vi "Is Already Exists.vi"(10 "Error":errorcluster) -> (2 "Error":errorcluster)   [LabVIEW 2020, in "jettl.lvlib" / "Actor.lvlib"]
uses:
  Actor.lvlib
  Error/Error.lvlib
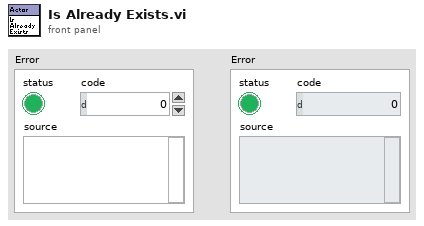
[diagram p1: front panel]
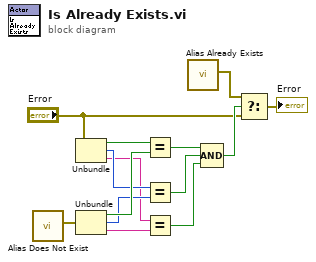
[diagram p0: block diagram]
diagram:
  n1 = call "Alias Does Not Exist.vi"() -> ("Error"=w14:errorcluster)  [unwired: 11 in]
  n2 = Unbundle("Error") -> ("status"=w13:bool, "code"=w11:i32, "source"=w9:string)
  n3 = Unbundle(w14) -> ("status"=w12:bool, "code"=w10:i32, "source"=w8:string)
  n4 = Equal?(x=w13, y=w12) -> (x = y?=w7:bool)
  n5 = Equal?(x=w11, y=w10) -> (x = y?=w6:bool)
  n6 = Equal?(x=w9, y=w8) -> (x = y?=w5:bool)
  n7 = call "Alias Already Exists.vi"() -> ("Error"=w2:errorcluster)  [unwired: 11 in]
  n8 = Compound Arithmetic op=AND(w7, w6, w5) -> (w4:bool)
  n9 = Select(t=w2, s=w4, f="Error") -> (s? t:f=→"Error":errorcluster)
